vi "OAT Polar PG Get Ready.vi"(6 "polar attributes":T2 {"minimum" format="%.2f"; "maximum" format="%.2f"}, 8 "rect":T5={"left"=0, "top"=0, "right"=324, "bottom"=234}, 9 "desired font(Application)":T3(ring)=enum."Application Font", 10 "[user-specified font]":T4) -> (5 "grid measurements":T1 {"end angle" format="%.2f"; "start angle" format="%.2f"; "scale factors"."b" format="%.2f"; "scale factors"."a" format="%.2f"}, 7 "decade specs":cluster{"radius":i16, "label":string}[](array[cluster]))   [LabVIEW 2017]
panel:
  in  "look up table":cluster{dbl, dbl}[](array[cluster])=[{0.0, 90.0}, {270.0, 360.0}, {180.0, 270.0}, {90.0, 180.0}, {0.0, 180.0}, {180.0, 360.0}, {270.0, 450.0}, {90.0, 270.0}, {0.0, 360.0}] {"?" format="%.2f"; "?" format="%.2f"}
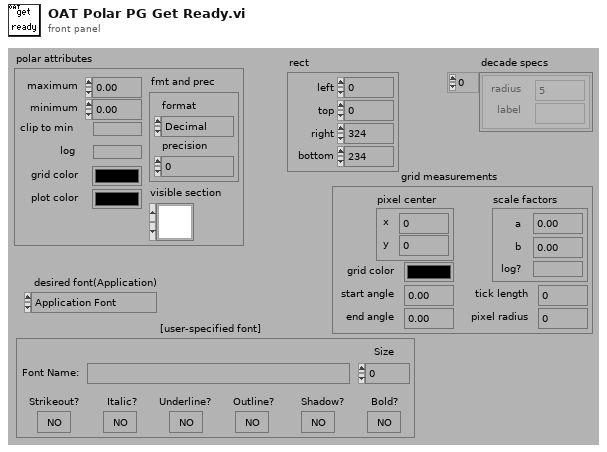
[diagram p1: front panel]
types:
  T1 = cluster{"pixel center":cluster{"x":i16, "y":i16}, "scale factors":cluster{"a":dbl, "b":dbl, "log?":bool}, "grid color":u32, "start angle":dbl, "end angle":dbl, "tick length":i16, "pixel radius":i32}
  T2 = cluster{"maximum":dbl, "minimum":dbl, "clip to min":bool, "log":bool, "grid color":u32, "plot color":u32, "fmt and prec":cluster{"format":enum8{"Decimal", "Scientific", "Engineering", "Binary", "Octal", "Hex"}, "precision":u8}, "visible section":u16}
  T3 = enum16{"User-specified Font", "Application Font", "System Font", "Dialog Font"}
  T4 = cluster{"Font Name:":string, "Size":i16, "Strikeout?":bool, "Italic?":bool, "Underline?":bool, "Outline?":bool, "Shadow?":bool, "Bold?":bool}
  T5 = cluster{"left":i16, "top":i16, "right":i16, "bottom":i16}
  T6 = cluster{"format":enum8{"Decimal", "Scientific", "Engineering", "Binary", "Octal", "Hex"}, "precision":u8}
  T7 = cluster{i32, "maximum":dbl, i32, "minimum":dbl, "log":bool, "fmt and prec":cluster{"format":enum8{"Decimal", "Scientific", "Engineering", "Binary", "Octal", "Hex"}, "precision":u8}}
  T8 = cluster{bool, bool, bool, "grid color":u32, "grid color":u32}
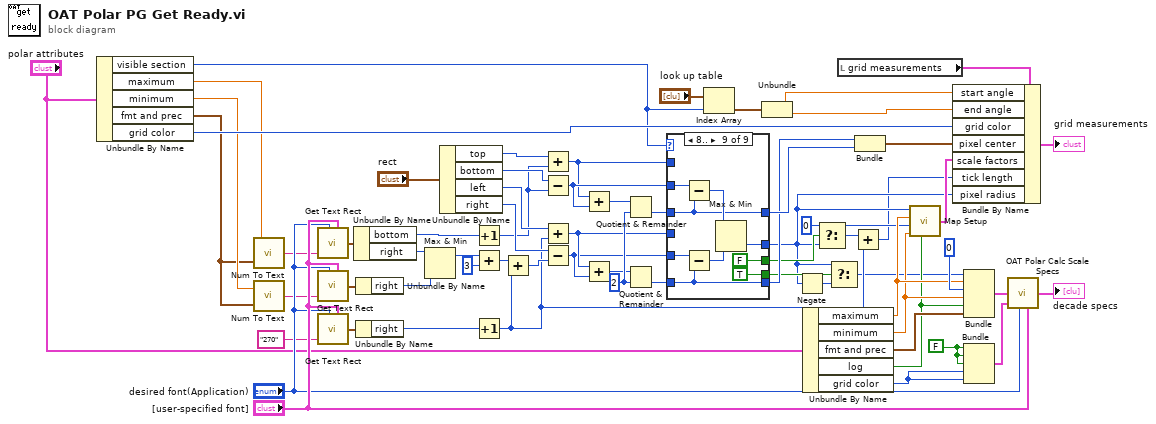
[diagram p0: block diagram]
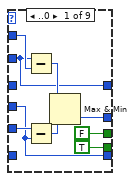
[diagram p2: hidden frame]
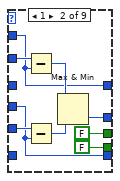
[diagram p3: hidden frame]
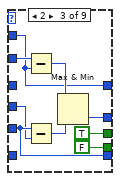
[diagram p4: hidden frame]
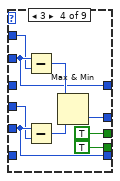
[diagram p5: hidden frame]
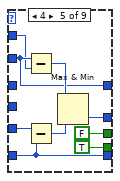
[diagram p6: hidden frame]
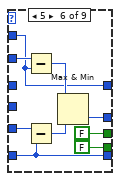
[diagram p7: hidden frame]
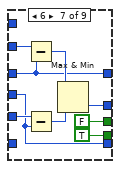
[diagram p8: hidden frame]
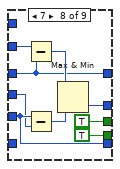
[diagram p9: hidden frame]
diagram:
  w13 = 0
  w1 = FALSE
  w59 = 2
  n1 = Unbundle By Name("polar attributes") -> ("visible section"=w9:u16, "maximum"=w32:dbl, "minimum"=w38:dbl, "fmt and prec"=w31:T6, "grid color"=w49:u32)
  n2 = call <vilib>:"Num To Text.vi"("fmt and prec"=w31, "number"=w32) -> ("numeric string"=w30:string)
  n3 = call <vilib>:"Num To Text.vi"("fmt and prec"=w31, "number"=w38) -> ("numeric string"=w56:string)
  n4 = call <vilib>:"Get Text Rect.vi"("desired font(Application)"="desired font(Application)", "text"=w30, "[user-specified font]"="[user-specified font]") -> ("rect"=w29:T5)  [unwired: 6 in]
  n5 = call <vilib>:"Get Text Rect.vi"("desired font(Application)"="desired font(Application)", "text"=w56, "[user-specified font]"="[user-specified font]") -> ("rect"=w55:T5)  [unwired: 6 in]
  n6 = call <vilib>:"Get Text Rect.vi"("desired font(Application)"="desired font(Application)", "text"="270", "[user-specified font]"="[user-specified font]") -> ("rect"=w54:T5)  [unwired: 6 in]
  n7 = Unbundle By Name(w29) -> ("bottom"=w26:i16, "right"=w28:i16)
  n8 = Unbundle By Name(w55) -> ("right"=w27:i16)
  n9 = Unbundle By Name(w54) -> ("right"=w24:i16)
  n10 = Max & Min(x=w28, y=w27) -> (max(x,y)=w10:i16)  [unwired: 1 out]
  n11 = Unbundle By Name("rect") -> ("top"=w63:i16, "bottom"=w62:i16, "left"=w61:i16, "right"=w60:i16)
  n12 = Increment(x=w26) -> (x+1=w25:i16)
  n13 = Add(x=w10, y=3) -> (x+y=w11:i32)
  n14 = Increment(x=w24) -> (x+1=w4:i16)
  n15 = Add(x=w11, y=w4) -> (x+y=w6:i32)
  n16 = Add(x=w63, y=w25) -> (x+y=w20:i16)
  n17 = Subtract(x=w62, y=w25) -> (x-y=w21:i16)
  n18 = Add(x=w61, y=w4) -> (x+y=w8:i16)
  n19 = Subtract(x=w60, y=w6) -> (x-y=w7:i32)
  n20 = Add(x=w20, y=w21) -> (x+y=w58:i16)
  n21 = Add(x=w8, y=w7) -> (x+y=w57:i32)
  n22 = Quotient & Remainder(x=w58, y=w59) -> (floor(x/y)=w19:i32)  [unwired: 1 out]
  n23 = Quotient & Remainder(x=w57, y=w59) -> (floor(x/y)=w22:i32)  [unwired: 1 out]
  n24 = case shown="8.." w9 {
    tunnel: w22 -> [_ _ _ _ w107 w114 _ _ w141]
    tunnel: w7 -> [w73 w81 w88 w98 w109 w117 w124 w133 w144]
    tunnel: w8 -> [w71 w79 w87 w96 _ _ w123 w132 _]
    tunnel: w19 -> [_ _ _ _ _ _ w125 w134 w142]
    tunnel: w21 -> [w69 w82 w91 w99 w106 w118 w127 w136 w145]
    tunnel: w20 -> [w70 w78 w89 w97 w105 w115 _ _ _]
    tunnel: [w72 w80 w90 w100 w108 w116 w126 w135 w143] -> w12
    tunnel: [w69 w78 w89 w99 w106 w115 w125 w134 w142] -> w18
    tunnel: [w71 w79 w88 w98 w107 w114 w123 w133 w141] -> w17
    tunnel: [TRUE FALSE FALSE TRUE TRUE FALSE TRUE TRUE TRUE] -> w16
    tunnel: [FALSE FALSE TRUE TRUE FALSE FALSE FALSE TRUE FALSE] -> w14
    frame ..0 {
      n25 = Subtract(x=w69, y=w70) -> (x-y=w74:i16)
      n26 = Subtract(x=w73, y=w71) -> (x-y=w75:i32)
      n27 = Max & Min(x=w74, y=w75) -> (min(x,y)=w72:i32)  [unwired: 1 out]
    }
    frame 1 {
      n28 = Subtract(x=w82, y=w78) -> (x-y=w83:i16)
      n29 = Subtract(x=w81, y=w79) -> (x-y=w84:i32)
      n30 = Max & Min(x=w83, y=w84) -> (min(x,y)=w80:i32)  [unwired: 1 out]
    }
    frame 2 {
      n31 = Subtract(x=w91, y=w89) -> (x-y=w92:i16)
      n32 = Subtract(x=w88, y=w87) -> (x-y=w93:i32)
      n33 = Max & Min(x=w92, y=w93) -> (min(x,y)=w90:i32)  [unwired: 1 out]
    }
    frame 3 {
      n34 = Subtract(x=w99, y=w97) -> (x-y=w101:i16)
      n35 = Subtract(x=w98, y=w96) -> (x-y=w102:i32)
      n36 = Max & Min(x=w101, y=w102) -> (min(x,y)=w100:i32)  [unwired: 1 out]
    }
    frame 4 {
      n37 = Subtract(x=w106, y=w105) -> (x-y=w110:i16)
      n38 = Subtract(x=w109, y=w107) -> (x-y=w111:i32)
      n39 = Max & Min(x=w110, y=w111) -> (min(x,y)=w108:i32)  [unwired: 1 out]
    }
    frame 5 {
      n40 = Subtract(x=w118, y=w115) -> (x-y=w119:i16)
      n41 = Subtract(x=w117, y=w114) -> (x-y=w120:i32)
      n42 = Max & Min(x=w119, y=w120) -> (min(x,y)=w116:i32)  [unwired: 1 out]
    }
    frame 6 {
      n43 = Subtract(x=w127, y=w125) -> (x-y=w128:i32)
      n44 = Subtract(x=w124, y=w123) -> (x-y=w129:i32)
      n45 = Max & Min(x=w128, y=w129) -> (min(x,y)=w126:i32)  [unwired: 1 out]
    }
    frame 7 {
      n46 = Subtract(x=w136, y=w134) -> (x-y=w137:i32)
      n47 = Subtract(x=w133, y=w132) -> (x-y=w138:i32)
      n48 = Max & Min(x=w137, y=w138) -> (min(x,y)=w135:i32)  [unwired: 1 out]
    }
    frame 8.. {
      n49 = Subtract(x=w145, y=w142) -> (x-y=w146:i32)
      n50 = Subtract(x=w144, y=w141) -> (x-y=w147:i32)
      n51 = Max & Min(x=w146, y=w147) -> (min(x,y)=w143:i32)  [unwired: 1 out]
    }
  }
  n52 = Index Array(array="look up table", index=w9) -> (element=w42:cluster{dbl, dbl})
  n53 = Unbundle(w42) -> (w40:dbl, w41:dbl)
  n54 = Negate(x=w12) -> (-x=w15:i32)
  n55 = Unbundle By Name("polar attributes") -> ("maximum"=w35:dbl, "minimum"=w34:dbl, "fmt and prec"=w39:T6, "log"=w33:bool, "grid color"=w46:u32)
  n56 = Select(t=w13, s=w14, f=w12) -> (s? t:f=w5:i32)
  n57 = Select(t=w12, s=w16, f=w15) -> (s? t:f=w2:i32)
  n58 = local read "grid measurements"() -> (w50:T1)
  n59 = Add(x=w5, y=w4) -> (x+y=w3:i32)
  n60 = Bundle(w17, w18) -> (w37:cluster{i32, i32})  [unwired: 1 in]
  n61 = call <vilib>:"Map Setup.vi"("coordinate 1"=w12, "value 1"=w35, "coordinate 2"=w13, "value 2"=w34, "log?(F)"=w33) -> ("scale factors"=w36:cluster{"a":dbl, "b":dbl, "log?(F)":bool})
  n62 = Bundle By Name(cluster=w50, "start angle"=w40, "end angle"=w41, "grid color"=w49, "pixel center"=w37, "scale factors"=w36, "tick length"=w3, "pixel radius"=w12) -> (→"grid measurements":T1)
  n63 = Bundle(w2, "maximum"=w35, 0, "minimum"=w34, "log"=w33, "fmt and prec"=w39) -> (w47:T7)  [unwired: 1 in]
  n64 = Bundle(w1, w1, w1, "grid color"=w46, "grid color"=w46) -> (w48:T8)  [unwired: 1 in]
  n65 = call <vilib>:"OAT Polar Calc Scale Specs.vi"("desired font(Application)"="desired font(Application)", "scale definition"=w47, "scale attributes"=w48, "[user-specified font]"="[user-specified font]") -> ("scale specs"=→"decade specs":cluster{"coordinate":i16, "label":string}[])  [unwired: 5 in]
